vi "Gaussian_PeakFitter.vi"(9 "Y array in":dbl[](array[numeric]), 10 "Peak Threshold":dbl format="%p", 11 "X array in":dbl[](array[numeric])) -> (1 "Amplitudes":dbl[](array[numeric]), 2 "peak detection locations":dbl[](array[numeric]), 3 "FWHM":dbl[](array[numeric]))   [LabVIEW 2016]
uses:
  <vilib>/Analysis/1siggen.llb/Ramp Pattern by Samples.vi
  <vilib>/Analysis/2dsp.llb/1D Convolution (DBL).vi
  <vilib>/Analysis/NI_AAL_SigProc.lvlib
  <vilib>/Analysis/NI_AALBase.lvlib
  <vilib>/Analysis/6fits.llb/Curve Fitting Criteria.ctl
  <vilib>/Analysis/NI_AALPro.lvlib
panel:
  out "FWHM start value":dbl[](array[numeric])
  out "FWHM end y value":dbl[](array[numeric])
  out "half peak amps":dbl[](array[numeric])
  out "FWHM start":dbl[](array[numeric])
  out "FWHM end":dbl[](array[numeric])
  out "some of the half-peak X values":dbl[](array[numeric])
  out "error":i32
  out "size original":i32
  out "size(s)":i32
  in  "peak fitting width":i32=3 min=3
  out "peak detection errors":i32
  in  "balance parameter":dbl=0.9999999 format="%#_20g"
  out "y size at the beginning":dbl
  out "spline error":i32
  in  "Smoothing Type":T1(ring)=enum."spline fit"
  out "raw in":cluster{"Y array":dbl[], "X array":dbl[]}(graph)
  out "Raw + Gaussians":T2(graph)
  out "X step":dbl
  out "best gassian fits":T2(graph)
  out "Gaussian Info Array":T3(array[cluster])
  out "Peak Detection Voltage Values":dbl[](array[numeric])
  out "smoothed":cluster{"Y array":dbl[], "X array":dbl[]}(graph)
  out "Y (out)":dbl[](array[numeric])
  out "X ramped (out)":dbl[](array[numeric])
  out "x size at beginnning":dbl
  out "Y size":i32
  out "X size":i32
  out "end":dbl
  out "start":dbl
  out "offset":dbl
  # "0.999999899999989394"
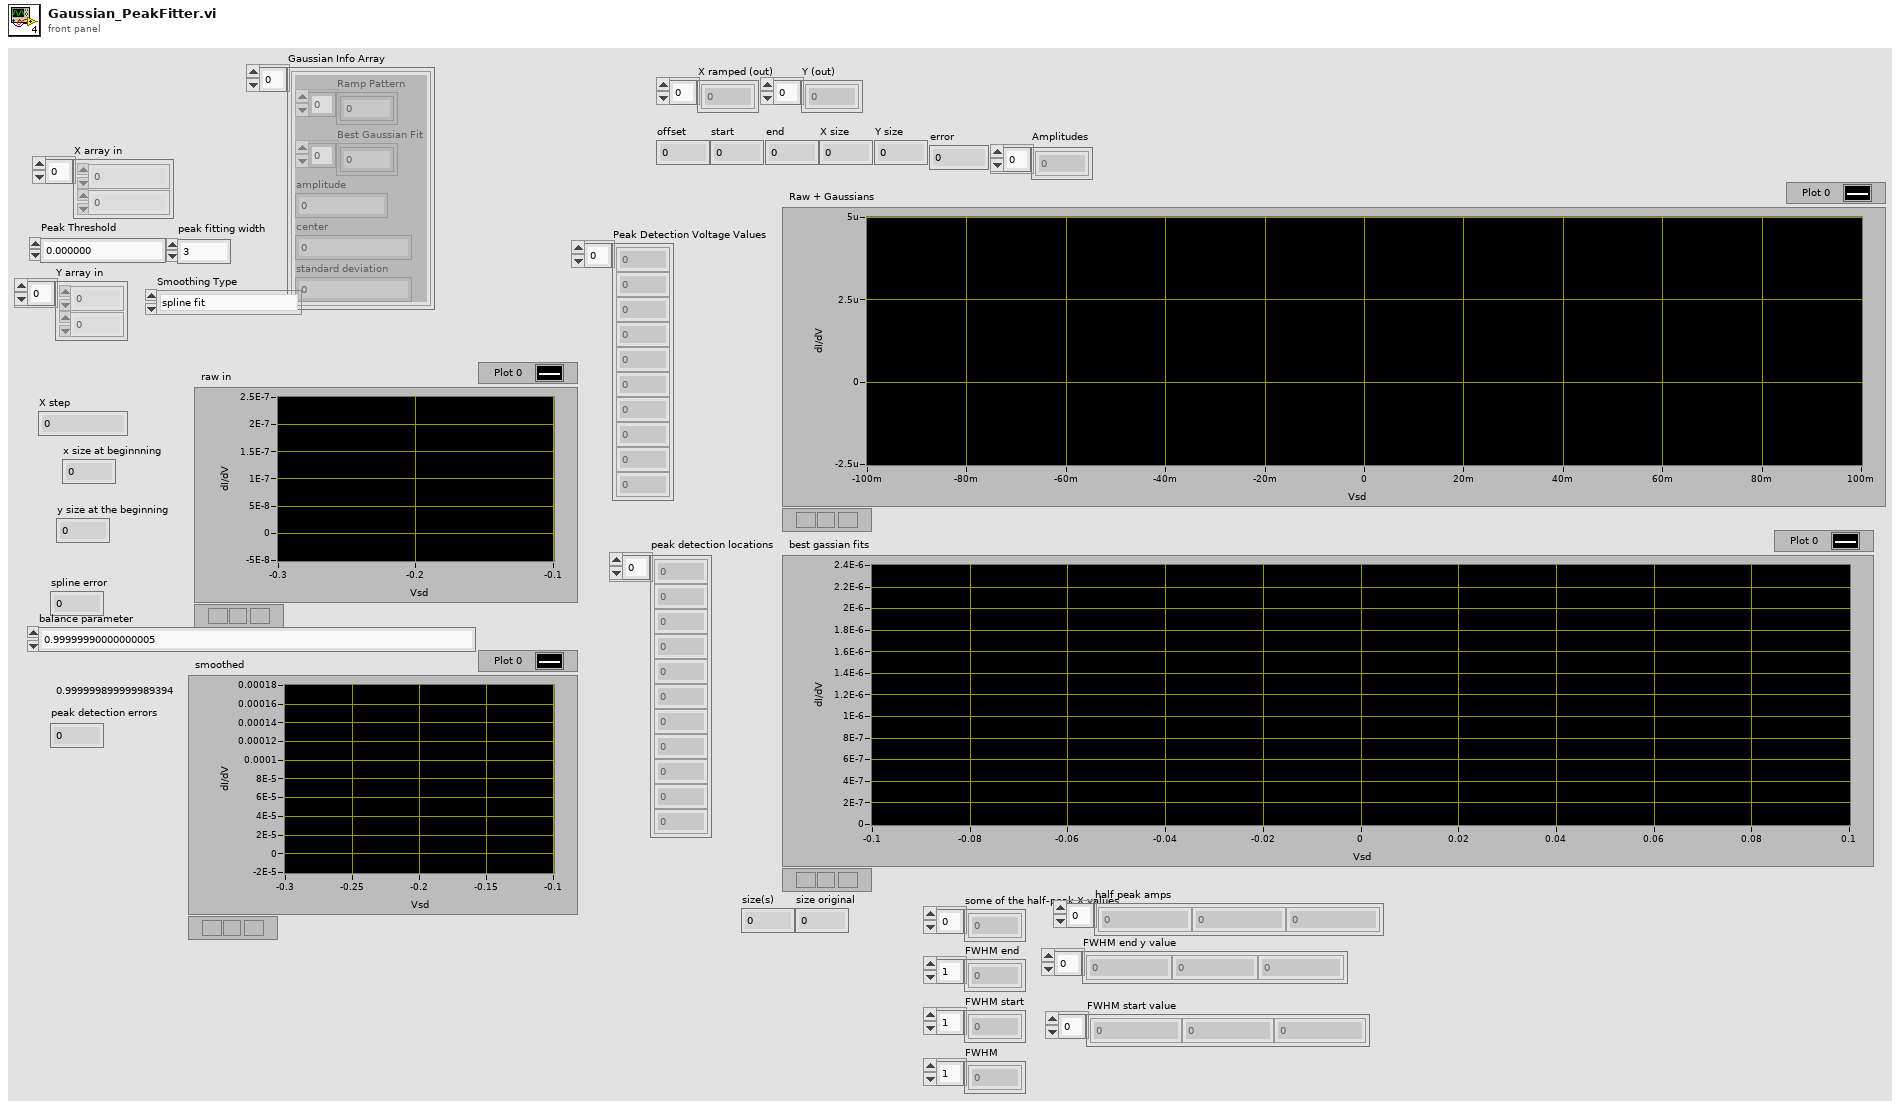
[diagram p1: front panel]
types:
  T1 = enum16{"none", "spline fit", "gaussian convolution"}
  T2 = cluster{"Ramp Pattern":dbl[], "Best Gaussian Fit":dbl[]}[]
  T3 = cluster{"Ramp Pattern":dbl[], "Best Gaussian Fit":dbl[], "amplitude":dbl, "center":dbl, "standard deviation":dbl}[]
  T4 = cluster{"amp min":dbl, "amp max":dbl, "center min":dbl, "center max":dbl, "deviation min":dbl, "deviation max":dbl, "offset min":dbl, "offset max":dbl}
  T5 = cluster{"initial amplitude":dbl, "initial center":dbl, "initial standard deviation":dbl, "offset":dbl}
  T6 = typedef "NI_AALPro.lvlib/Curve Fitting Criteria.ctl" = u16
  T7 = cluster{"Ramp Pattern":dbl[], "Best Gaussian Fit":dbl[], "amplitude":dbl, "center":dbl, "standard deviation":dbl}
  T8 = cluster{"Ramp Pattern":dbl[], "Best Gaussian Fit":dbl[]}
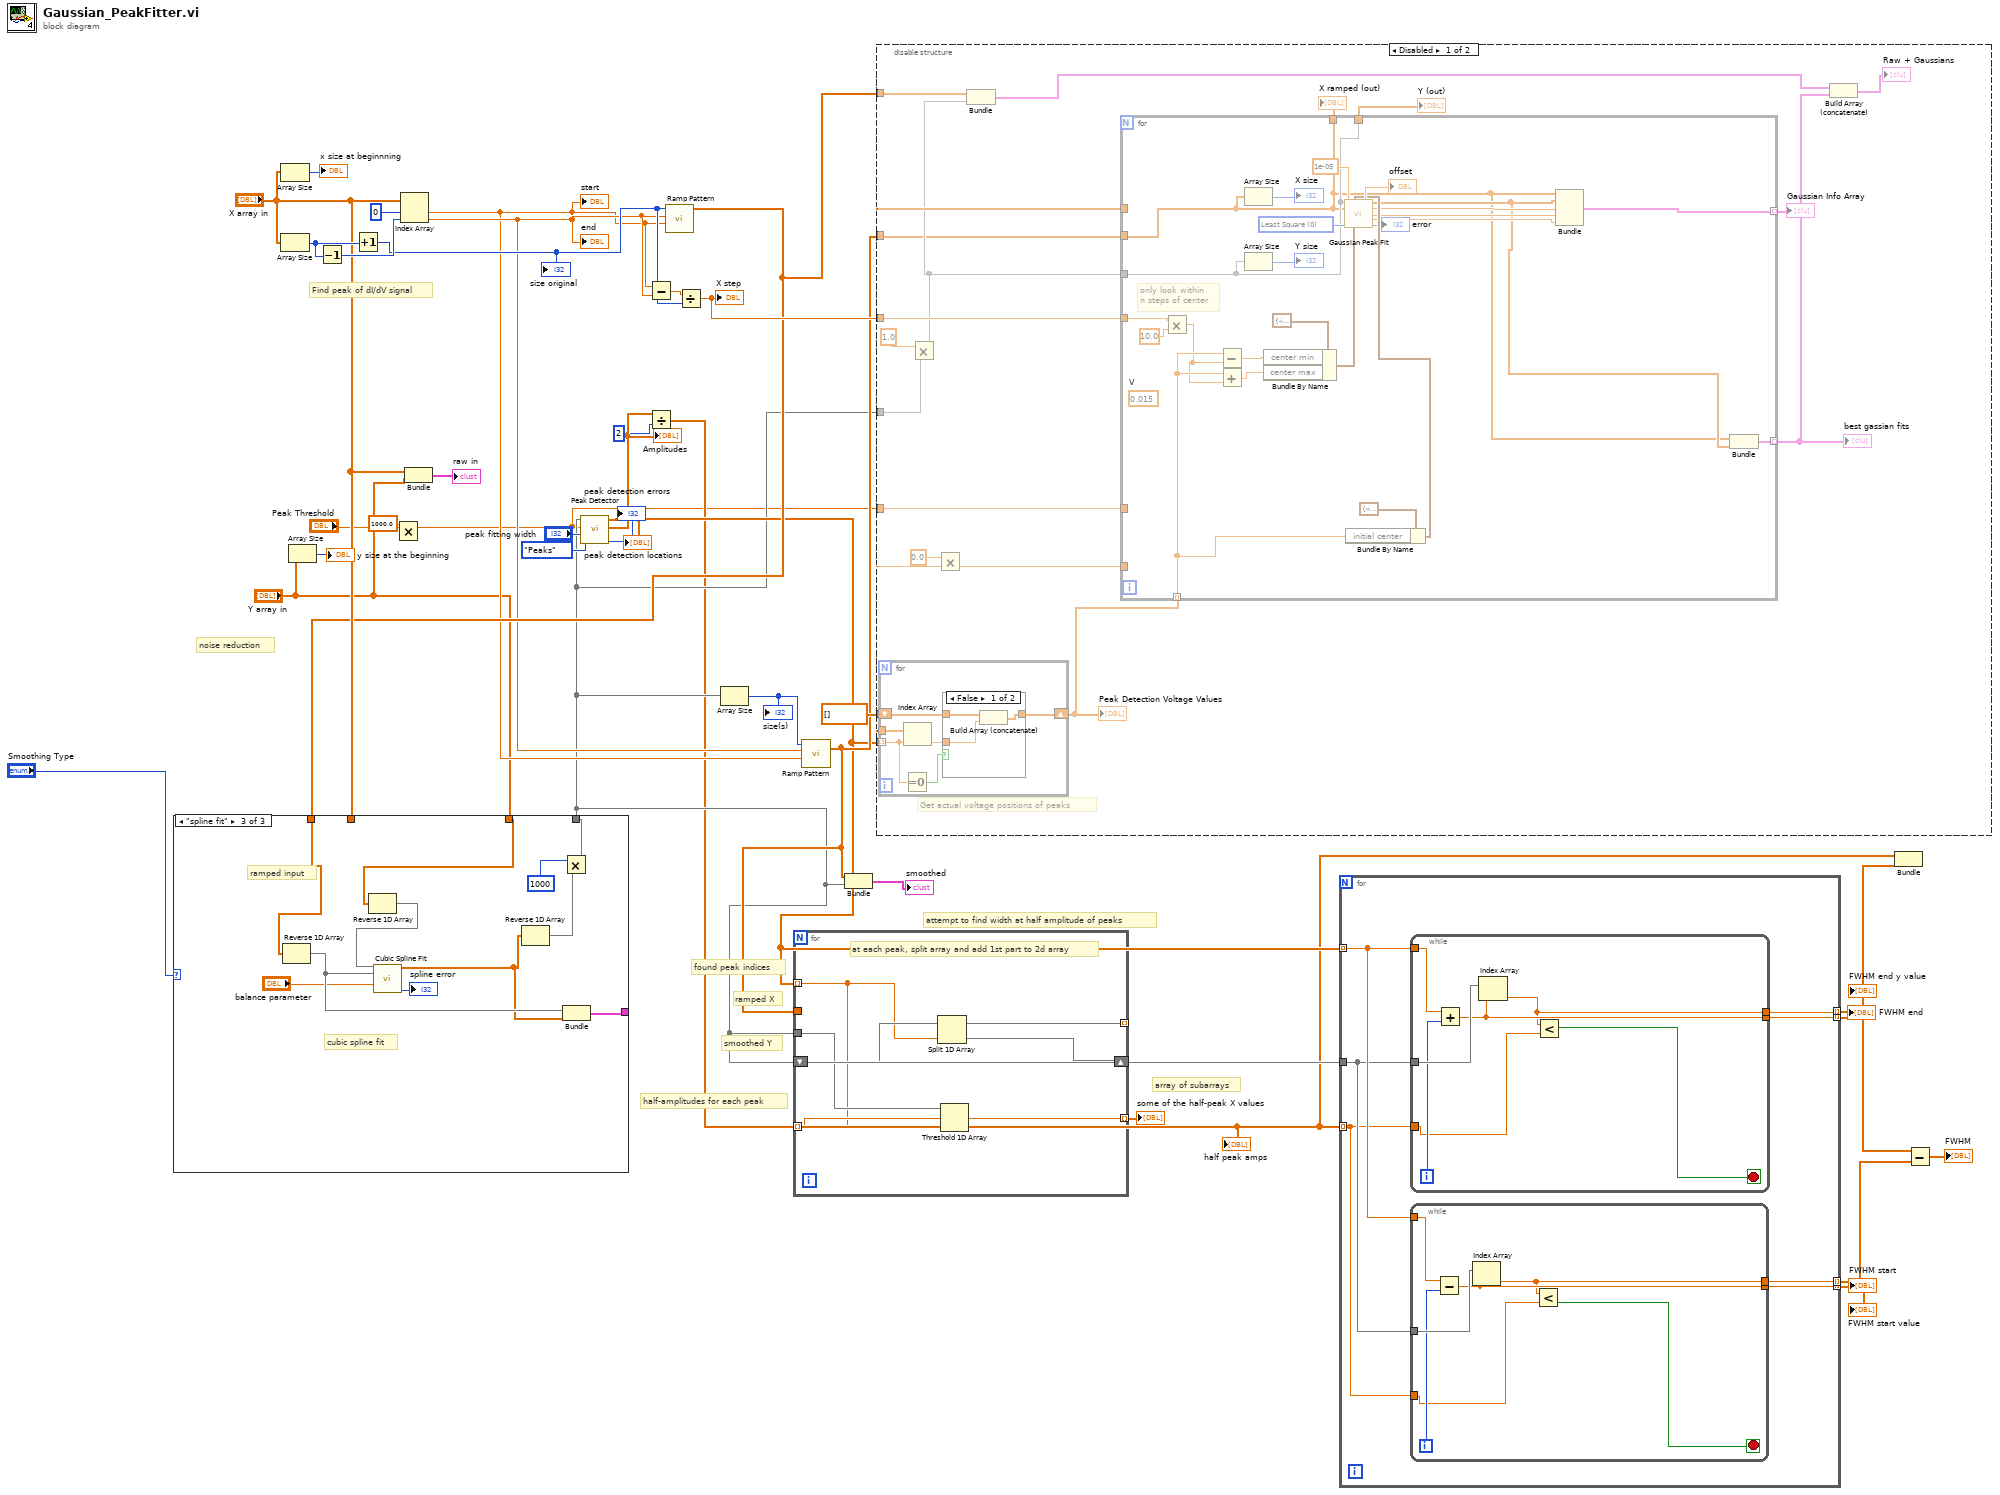
[diagram p0: block diagram]
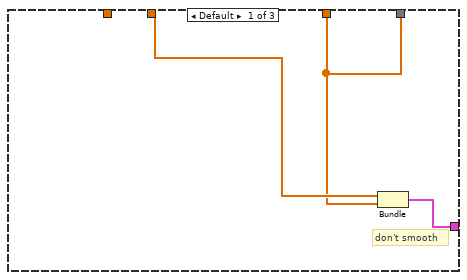
[diagram p4: hidden frame]
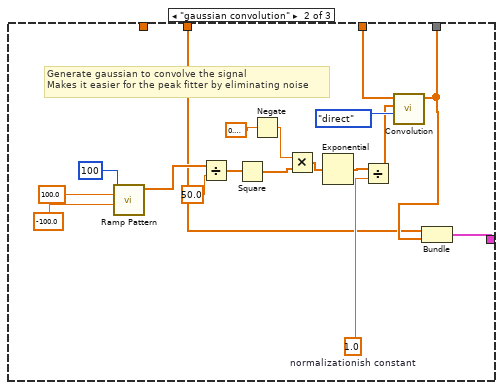
[diagram p5: hidden frame]
diagram:
  # "half-amplitudes for each peak"
  # "array of subarrays"
  # "found peak indices"
  # "ramped X"
  # "smoothed Y"
  # "attempt to find width at half amplitude of peaks"
  # "noise reduction"
  # "Find peak of dI/dV signal"
  n1 = Array Size(array="X array in") -> (size(s)=→"x size at beginnning":i32)
  n2 = Array Size(array="X array in") -> (size(s)=w35:i32)
  n3 = Array Size(array="Y array in") -> (size(s)=→"y size at the beginning":i32)
  n4 = Decrement(x=w35) -> (x-1=w34:i32)
  n5 = Increment(x=w35) -> (x+1=w31:i32)
  "size original" <- w31
  n6 = Multiply(x="Peak Threshold", y=1000.0) -> (x*y=w2:dbl)
  n7 = Index Array(array="X array in", index #1=0 ("index"), index #2=w34) -> (element #1=w19:dbl, element #2=w20:dbl)
  "start" <- w19
  "end" <- w20
  n8 = Bundle("X array in"="X array in", "Y array in"="Y array in") -> (→"raw in":cluster{"X array in":dbl[], "Y array in":dbl[]})  [unwired: 1 in]
  n9 = Subtract(x=w19, y=w20) -> (x-y=w30:dbl)
  n10 = call-poly <vilib>:"Ramp Pattern.vi"("start"=w19, "end"=w20, "samples"=w31) -> ("Ramp Pattern"=w24:dbl[])  [unwired: 7 in, 1 out]
  n11 = case shown="\"spline fit\"" "Smoothing Type" {
    tunnel: [w38 w47 w59] -> w7
    tunnel: [w37 w45 w68] -> _
    tunnel: "X array in" -> [w39 w41 _]
    tunnel: "Y array in" -> [w38 w40 w66]
    tunnel: w24 -> [_ _ w64]
    frame Default {
      # "don't smooth"
      n12 = Bundle("X array in"=w39, "Y array in"=w38) -> (w37:cluster{"X array in":dbl[], "Y array in":dbl[]})  [unwired: 1 in]
    }
    frame "gaussian convolution" {
      w42 = 1.0  # normalizationish constant
      # "Generate gaussian to convolve the signal\nMakes it easier for the peak fitter by eliminating noise"
      n13 = call-poly <vilib>:"Ramp Pattern.vi"("start"=-100.0, "end"=100.0, "samples"=100) -> ("Ramp Pattern"=w54:dbl[])  [unwired: 7 in, 1 out]
      n14 = Divide(x=w54, y=50.0 ("end")) -> (x/y=w52:dbl[])
      n15 = Square(x=w52) -> (x^2=w51:dbl[])
      n16 = Negate(x=0.6931471805599453) -> (-x=w50:dbl)
      n17 = Multiply(x=w50, y=w51) -> (x*y=w48:dbl[])
      n18 = Exponential(1:w48) -> (0:w43:dbl[])
      n19 = Divide(x=w43, y=w42) -> (x/y=w44:dbl[])
      n20 = call-poly <vilib>:"Convolution.vi"("algorithm"=enum32{"direct", "frequency domain"}."direct", "Y"=w44, "X"=w40) -> ("X * Y"=w47:dbl[])  [unwired: 7 in, 1 out]
      n21 = Bundle("X array in"=w41, "X * Y"=w47) -> (w45:cluster{"X array in":dbl[], "X * Y":dbl[]})  [unwired: 1 in]
    }
    frame "spline fit" {
      # "ramped input"
      # "cubic spline fit"
      n22 = Reverse 1D Array(array=w64) -> (reversed array=w63:dbl[])
      n23 = Reverse 1D Array(array=w66) -> (reversed array=w65:dbl[])
      n24 = call <vilib>:"Cubic Spline Fit.vi"("Y"=w65, "X"=w63, "balance parameter"="balance parameter") -> ("Best Cubic Spline Fit"=w60:dbl[], "error"=→"spline error":i32)  [unwired: 11 in]
      n25 = Reverse 1D Array(array=w60) -> (reversed array=w61:dbl[])
      n26 = Multiply(x=1000, y=w61) -> (x*y=w59:dbl[])
      n27 = Bundle(w63, "Best Cubic Spline Fit"=w60) -> (w68:cluster{dbl[], "Best Cubic Spline Fit":dbl[]})  [unwired: 1 in]
    }
  }
  n28 = call <vilib>:"Peak Detector.vi"("peaks/valleys"=enum32{"Peaks", "Valleys"}."Peaks", "width"="peak fitting width", "threshold"=w2, "X"=w7) -> ("error"=→"peak detection errors":i32, "Amplitudes"=w14:dbl[], "Locations"=w10:dbl[])  [unwired: 3 in, 2 out]
  "peak detection locations" <- w10
  "Amplitudes" <- w14
  n29 = Divide(x=w14, y=2) -> (x/y=w6:dbl[])
  "half peak amps" <- w6
  n30 = Divide(x=w30, y=w31) -> (x/y=w29:dbl)
  "X step" <- w29
  n31 = Array Size(array=w7) -> (size(s)=w18:i32)
  "size(s)" <- w18
  n32 = call-poly <vilib>:"Ramp Pattern.vi"("start"=w19, "end"=w20, "samples"=w18) -> ("Ramp Pattern"=w12:dbl[])  [unwired: 7 in, 1 out]
  n33 = for {
    tunnel: w7 -> [w72]
    tunnel: w12 -> [_]
    tunnel: w10 -> [w70] mode=indexing
    shift-right: [w74] -> _
    shift-left: w7 -> [w73]
    tunnel: [w75] -> _ mode=indexing
    tunnel: w6 -> [w71] mode=indexing
    tunnel: [w69] -> w11 mode=indexing
    # "at each peak, split array and add 1st part to 2d array"
    n34 = Split 1D Array(array=w73, index=w70) -> (first subarray=w75:dbl[], second subarray=w74:dbl[])
    n35 = Threshold 1D Array(1:w70, 2:w71, 3:w72) -> (0:w69:dbl)
  }
  "some of the half-peak X values" <- w11
  n36 = Bundle("Ramp Pattern"=w12, "X * Y"=w7) -> (→"smoothed":cluster{"Ramp Pattern":dbl[], "X * Y":dbl[]})  [unwired: 1 in]
  n37 = disable-structure shown="Disabled" {
    disable-tunnel: dbl[] [] -> [w91 _]
    disable-tunnel: w29 -> [w88 _]
    disable-tunnel: w24 -> [w84 _]
    disable-tunnel: w2 -> [w81 _]
    disable-tunnel: w12 -> [w78 _]
    disable-tunnel: w10 -> [w77 _]
    disable-tunnel: w7 -> [w76 _]
    frame Disabled {
      # "Get actual voltage positions of peaks"
      n38 = for {
        tunnel: w77 -> [w96] mode=indexing
        shift-right: [w94] -> w90
        shift-left: w91 -> [w99]
        tunnel: w78 -> [w98]
        n39 = Equal To 0?(x=w96) -> (x = 0?=w95:bool)
        n40 = Index Array(array=w98, index=w96) -> (element=w97:dbl)
        n41 = case shown="False" w95 {
          tunnel: [w102 w103] -> w94
          tunnel: w99 -> [w101 w103]
          tunnel: w97 -> [w100 _]
          frame False {
            n42 = Build Array (concatenate)(w101, w100) -> (w102:dbl[])
          }
          frame True {
          }
        }
      }
      "Peak Detection Voltage Values" <- w90
      n43 = Multiply(x=1.0, y=w76) -> (x*y=w83:dbl[])
      n44 = Multiply(x=0.0, y=w81) -> (x*y=w80:dbl)
      n45 = Bundle("Ramp Pattern"=w84, w83) -> (w87:cluster{"Ramp Pattern":dbl[], dbl[]})  [unwired: 1 in]
      n46 = for {
        tunnel: w83 -> [w107]
        tunnel: w84 -> [_]
        tunnel: w81 -> [_]
        tunnel: [w104] -> w93
        tunnel: [w107] -> w92
        tunnel: w90 -> [w110] mode=indexing
        tunnel: [w118] -> w89 mode=indexing
        tunnel: [w117] -> w85 mode=indexing
        tunnel: w88 -> [w113]
        tunnel: w80 -> [_]
        tunnel: w78 -> [w104]
        (unwired) 0.015  # V
        w126 = T6 0 items=["Least Square", "Least Absolute Residual", "Bisquare"] ("method")
        # "only look within\nn steps of center"
        n47 = Multiply(x=w113, y=10.0) -> (x*y=w109:dbl)
        n48 = Subtract(x=w110, y=w109) -> (x-y=w112:dbl)
        n49 = Add(x=w110, y=w109) -> (x+y=w111:dbl)
        n50 = Array Size(array=w104) -> (size(s)=→"X size":i32)
        n51 = Array Size(array=w107) -> (size(s)=→"Y size":i32)
        n52 = Bundle By Name(cluster=T4 {"amp min"=-inf, "amp max"=inf, "center min"=-inf, "center max"=inf, "deviation min"=-inf, "deviation max"=inf, "offset min"=0.0, "offset max"=0.0} ("parameter bounds"), "center min"=w112, "center max"=w111) -> (w106:T4)
        n53 = Bundle By Name(cluster=T5 {"initial amplitude"=nan, "initial center"=nan, "initial standard deviation"=nan, "offset"=nan} ("initial guess"), "initial center"=w110) -> (w122:T5)
        n54 = call <vilib>:"Gaussian Peak Fit.vi"("Y"=w107, "initial guess"=w122, "X"=w104, "tolerance"=1e-05, "method"=w126, "parameter bounds"=w106) -> ("offset"=→"offset":dbl, "Best Gaussian Fit"=w116:dbl[], "amplitude"=w121:dbl, "center"=w120:dbl, "standard deviation"=w119:dbl, "error"=→"error":i32)  [unwired: 3 in, 1 out]
        n55 = Bundle("Ramp Pattern"=w104, "Best Gaussian Fit"=w116, "amplitude"=w121, "center"=w120, "standard deviation"=w119) -> (w118:T7)  [unwired: 1 in]
        n56 = Bundle("Ramp Pattern"=w104, "Best Gaussian Fit"=w116) -> (w117:T8)  [unwired: 1 in]
      }
      "X ramped (out)" <- w93
      "Y (out)" <- w92
      "Gaussian Info Array" <- w89
      "best gassian fits" <- w85
      n57 = Build Array (concatenate)(w87, w85) -> (→"Raw + Gaussians":T2)
    }
    frame Enabled {
    }
  }
  n58 = for {
    tunnel: w7 -> [w132]
    tunnel: w6 -> [w131] mode=indexing
    tunnel: w10 -> [w133] mode=indexing
    tunnel: [w134] -> w5 mode=indexing
    tunnel: [w130] -> w9 mode=indexing
    tunnel: [w129] -> w4 mode=indexing
    tunnel: [w128] -> w3 mode=indexing
    n59 = while {
      tunnel: w132 -> [w141]
      tunnel: w131 -> [w138]
      tunnel: w133 -> [w140]
      tunnel: [w136] -> w130
      tunnel: [w135] -> w128
      i -> [w139]
      stop <- w137 stop-if-true
      n60 = Subtract(x=w140, y=w139) -> (x-y=w136:dbl)
      n61 = Index Array(array=w141, index=w136) -> (element=w135:dbl)
      n62 = Less?(x=w135, y=w138) -> (x < y?=w137:bool)
    }
    n63 = while {
      tunnel: w132 -> [w148]
      tunnel: w131 -> [w145]
      tunnel: w133 -> [w147]
      tunnel: [w143] -> w134
      tunnel: [w142] -> w129
      i -> [w146]
      stop <- w144 stop-if-true
      n64 = Add(x=w147, y=w146) -> (x+y=w143:dbl)
      n65 = Index Array(array=w148, index=w143) -> (element=w142:dbl)
      n66 = Less?(x=w142, y=w145) -> (x < y?=w144:bool)
    }
  }
  "FWHM end" <- w5
  "FWHM start" <- w9
  "FWHM end y value" <- w4
  "FWHM start value" <- w3
  n67 = Bundle(w6, w5) -> ()  [unwired: 1 in, 1 out]
  n68 = Subtract(x=w5, y=w9) -> (x-y=→"FWHM":dbl[])
